vi "串口读取.vi"() -> ()   [LabVIEW 2020]
uses:
  <vilib>/Instr/_visa.llb/VISA Configure Serial Port (Instr).vi
panel:
  out "数组 3":sgl[](array[numeric])
  out "数组":string[](array[string])
  out "数组 2":i32[](array[numeric])
  out "读取缓冲区":string
  in  "VISA resource name":refnum<visa-resource-name> caption="VISA资源名称"
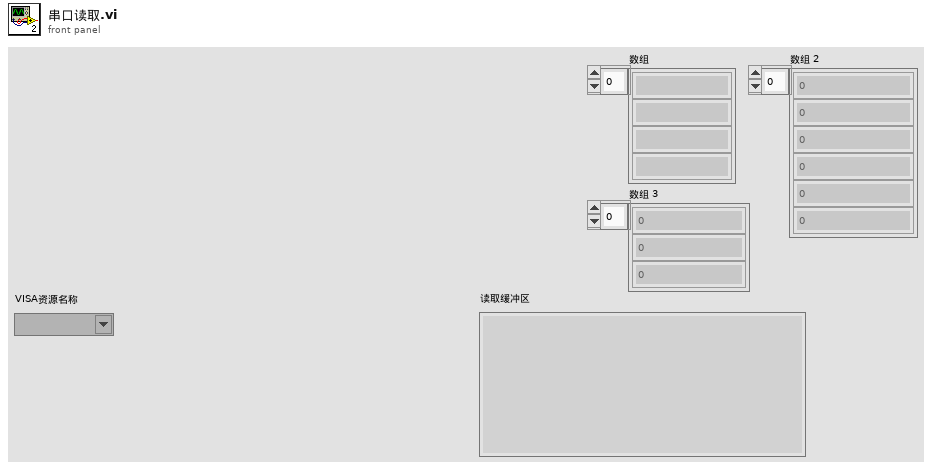
[diagram p1: front panel]
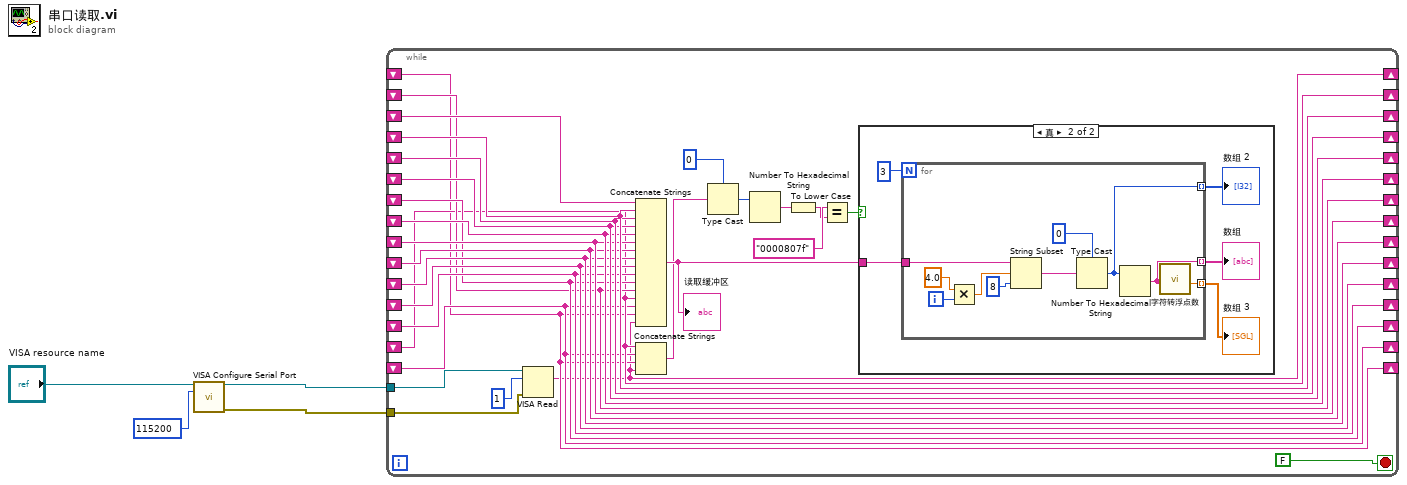
[diagram p0: block diagram]
diagram:
  n1 = call-poly "VISA Configure Serial Port"("VISA resource name"="VISA resource name", "baud rate (9600)"=u32 115200) -> ("VISA resource name out"=w2:refnum<visa-resource-name>, "error out"=w1:errorcluster)  [unwired: 12 in]
  n2 = while {
    tunnel: w2 -> [w30]
    tunnel: w1 -> [w29]
    shift-right: [w14] -> _
    shift-left: _ -> [w15]
    shift-right: [w15] -> _
    shift-left: _ -> [w16]
    shift-right: [w16] -> _
    shift-left: _ -> [w17]
    shift-right: [w17] -> _
    shift-left: _ -> [w18]
    shift-right: [w18] -> _
    shift-left: _ -> [w19]
    shift-right: [w19] -> _
    shift-left: _ -> [w20]
    shift-right: [w20] -> _
    shift-left: _ -> [w21]
    shift-right: [w21] -> _
    shift-left: _ -> [w22]
    shift-right: [w22] -> _
    shift-left: _ -> [w23]
    shift-right: [w23] -> _
    shift-left: _ -> [w24]
    shift-right: [w24] -> _
    shift-left: _ -> [w25]
    shift-right: [w10] -> _
    shift-left: _ -> [w11]
    shift-right: [w11] -> _
    shift-left: _ -> [w12]
    shift-right: [w12] -> _
    shift-left: _ -> [w13]
    shift-right: [w13] -> _
    shift-left: _ -> [w14]
    stop <- FALSE stop-if-true
    n3 = VISA Read(VISA resource name=w30, byte count=u32 1 ("字节总数"), error in (no error)=w29) -> (read buffer=w10:string)  [unwired: 3 out]
    n4 = Concatenate Strings(w25, w24, w23, w22, w21, w20, w19, w18, w17, w16, w15, w14, w13, w12, w11, w10) -> (w9:string)
    "读取缓冲区" <- w9
    n5 = Concatenate Strings(w13, w12, w11, w10) -> (w8:string)
    n6 = Type Cast(type=0 ("长度（剩余）"), x=w8) -> (*(type *) &x=w6:i32)
    n7 = Number To Hexadecimal String(2:w6) -> (0:w5:string)  [unwired: 1 in]
    n8 = To Lower Case(string=w5) -> (all lower case string=w27:string)
    n9 = Equal?(x="0000807f" ("y"), y=w27) -> (x = y?=w26:bool)
    n10 = case shown="真" w26 {
      tunnel: w9 -> [_ w33]
      frame False {
      }
      frame True {
        n11 = for {
          N: 3 -> [_]
          tunnel: [w42] -> w37 mode=indexing
          tunnel: [w41] -> w36 mode=indexing
          tunnel: [w40] -> w35 mode=indexing
          tunnel: w33 -> [w38]
          i -> [w46]
          n12 = Multiply(x=4.0, y=w46) -> (x*y=w45:dbl)
          n13 = String Subset(string=w38, offset (0)=w45, length (rest)=8 ("长度（剩余）")) -> (substring=w39:string)
          n14 = Type Cast(type=0 ("长度（剩余）"), x=w39) -> (*(type *) &x=w42:i32)
          n15 = Number To Hexadecimal String(2:w42) -> (0:w41:string)  [unwired: 1 in]
          n16 = call "字符转浮点数.vi"("十六进制32bit"=w41) -> ("数值"=w40:sgl)  [unwired: 10 in]
        }
        "数组 2" <- w37
        "数组" <- w36
        "数组 3" <- w35
      }
    }
  }
